vi "DrawScore.vi"(5 "Digits":i32, 6 "AutoWidth?":bool, 7 "Color":T2, 8 "error in (no error)":errorcluster, 9 "score":i16, 10 "position":T1) -> (0 "error out":errorcluster)   [LabVIEW 2019, in "RT_Game.lvlib" / "Engine.lvclass"]
uses:
  Engine.lvclass
  Color.ctl
  Coordinate.ctl
  RT_Game.lvlib
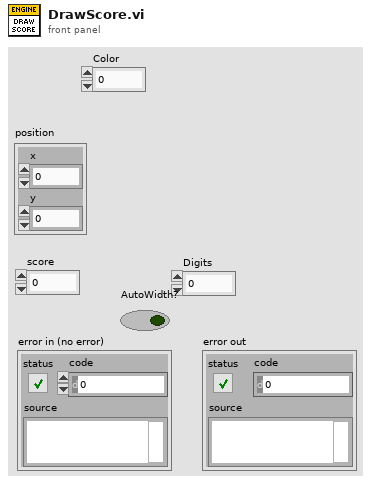
[diagram p1: front panel]
types:
  T1 = typedef "RT_Game.lvlib/Engine.lvclass/Coordinate.ctl" = cluster{"x":dbl, "y":dbl}
  T2 = typedef "RT_Game.lvlib/Color.ctl" = fxp<+,3,3>
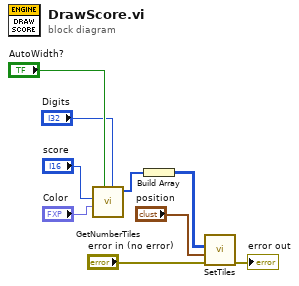
[diagram p0: block diagram]
diagram:
  n1 = call "GetNumberTiles.vi"("Digits"="Digits", "AutoWidth? (f)"="AutoWidth?", "Color"="Color", "score"="score") -> ("Tiles"=w8:u32[])  [unwired: 7 in]
  n2 = Build Array(w8) -> (w9:u32[][])
  n3 = call "SetTiles.vi"("error in (no error)"="error in (no error)", "Position"="position", "TileCodes"=w9) -> ("error out"=→"error out":errorcluster)  [unwired: 8 in]
